vi "Check Handle.vi"(8 "error in (no error)":errorcluster, 9 "Array":refnum<k15>[](array[refnum]), 10 "Connection Array":T1, 11 "Handle In":string) -> (0 "error out":errorcluster, 2 "Duplicate Instrument?":bool, 3 "Handle Out":string)   [LabVIEW 2018, in "ScopePlugins.lvlib" / "ScopePluginsBase.lvclass"]
uses:
  ScopePluginsBase.lvclass
  NIScopeClass/PublicMethods/ConnectionArray.ctl
  NIScopeClass/NIScope.lvclass
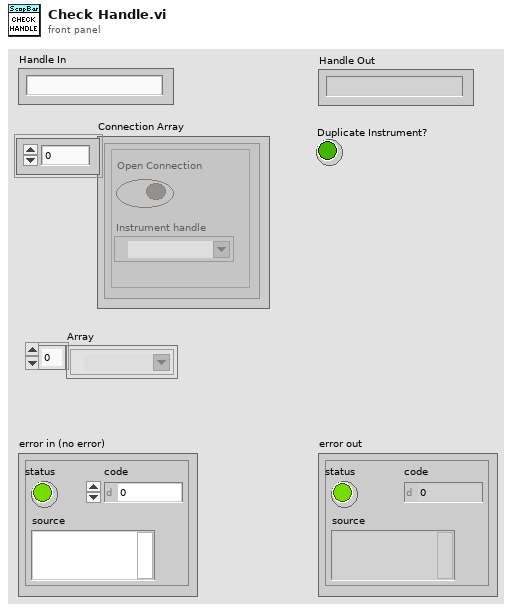
[diagram p1: front panel]
types:
  T1 = typedef "ScopePlugins.lvlib/NIScope.lvclass/ConnectionArray.ctl" = cluster{"Open Connection":bool, "Instrument handle":refnum<k15>}[]
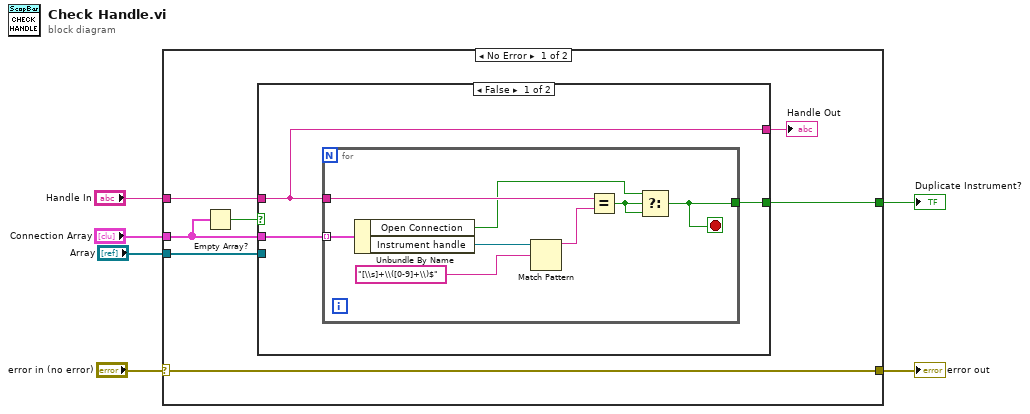
[diagram p0: block diagram]
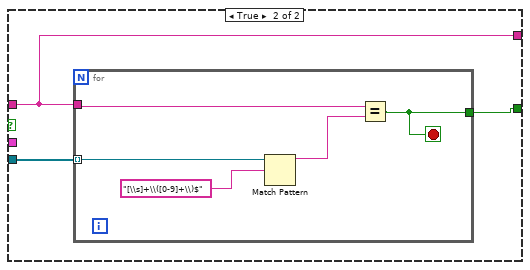
[diagram p2: hidden frame]
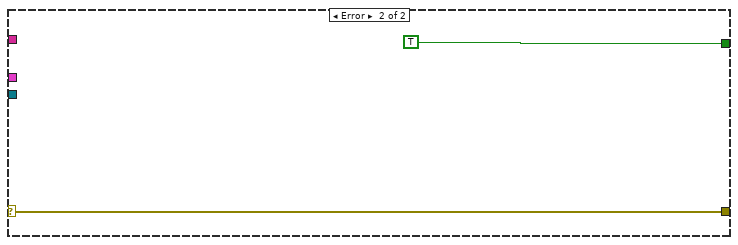
[diagram p3: hidden frame]
diagram:
  n1 = case shown="No Error" "error in (no error)" {
    selector: "error in (no error)" -> [w13 w34]
    tunnel: [w13 w34] -> w5
    tunnel: "Connection Array" -> [w8 _]
    tunnel: "Handle In" -> [w12 _]
    tunnel: [w9 TRUE] -> w3
    tunnel: "Array" -> [w11 _]
    frame No Error {
      n2 = Empty Array?(array=w8) -> (empty?=w7:bool)
      n3 = case shown="False" w7 {
        tunnel: w12 -> [w14 w25]
        tunnel: [w16 w27] -> w9
        tunnel: w8 -> [w15 _]
        tunnel: w11 -> [_ w26]
        tunnel: [w14 w25] -> w10
        frame False {
          n4 = for {
            tunnel: w14 -> [w22]
            tunnel: [w21] -> w16
            tunnel: w15 -> [w20] mode=indexing
            stop <- w21 stop-if-true
            n5 = Unbundle By Name(w20) -> ("Open Connection"=w19:bool, "Instrument handle"=w17:refnum<k15>)
            n6 = Match Pattern(string=w17, regular expression="[\\s]+\\([0-9]+\\)$") -> (before substring=w23:string)  [unwired: 1 in, 3 out]
            n7 = Equal?(x=w22, y=w23) -> (x = y?=w18:bool)
            n8 = Select(t=w19, s=w18, f=w18) -> (s? t:f=w21:bool)
          }
        }
        frame True {
          n9 = for {
            tunnel: w25 -> [w29]
            tunnel: [w30] -> w27
            tunnel: w26 -> [w28] mode=indexing
            stop <- w30 stop-if-true
            n10 = Match Pattern(string=w28, regular expression="[\\s]+\\([0-9]+\\)$") -> (before substring=w32:string)  [unwired: 1 in, 3 out]
            n11 = Equal?(x=w29, y=w32) -> (x = y?=w30:bool)
          }
        }
      }
      "Handle Out" <- w10
    }
    frame Error {
    }
  }
  "error out" <- w5
  "Duplicate Instrument?" <- w3
